vi "get_comments_experiment_group.vi"(0 "Experiments_group.lvclass in":refnum<class "Experiments_group.lvclass">, 1 "error in (no error)":errorcluster) -> (2 "Comments":string, 3 "Experiments_group.lvclass out":refnum<class "Experiments_group.lvclass">, 4 "error out":errorcluster)   [LabVIEW 2019, in "Experiments_group.lvclass"]
uses:
  Experiments_group.lvclass
  Experiments_group.lvclass/Experiments_group.ctl
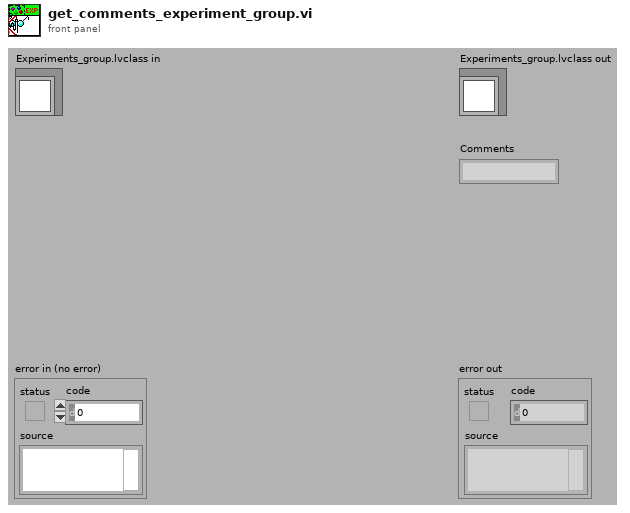
[diagram p1: front panel]
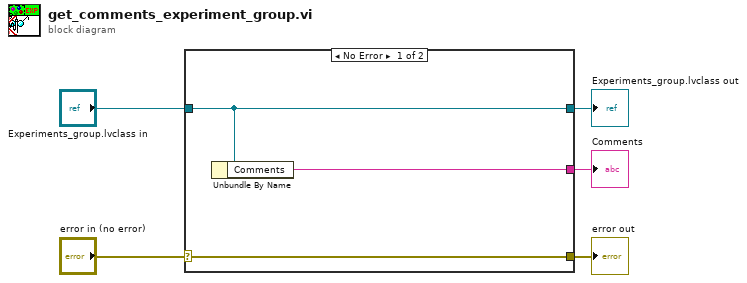
[diagram p0: block diagram]
diagram:
  n1 = case shown="No Error" "error in (no error)" {
    selector: "error in (no error)" -> [w8 w9]
    tunnel: [w8 w9] -> w4
    tunnel: [w7 w10] -> w2
    tunnel: "Experiments_group.lvclass in" -> [w7 w10]
    tunnel: [w6 _] -> w1
    frame No Error {
      n2 = Unbundle By Name(w7) -> ("Comments"=w6:string)
    }
    frame Error {
    }
  }
  "error out" <- w4
  "Experiments_group.lvclass out" <- w2
  "Comments" <- w1
